vi "initalize delta(SubVI).vi"(9 "字符串":string, 11 "队列输出":refnum<queue>) -> ()   [LabVIEW 2019, in "SubVI.lvlib"]
uses:
  SubVI.lvlib
  lib/Keithley 622x/Configure/Delta PDelta DCon Modes/Typedefs/KE622x -- Delta Mode Params.ctl
  lib/Keithley 622x/Configure/Delta PDelta DCon Modes/Low Level/Typedefs/KE622x -- Delta PDelta Mode High Level.ctl
  lib/Keithley 622x/Configure/Delta PDelta DCon Modes/Low Level/Typedefs/KE622x -- Delta PDelta Mode Low Level.ctl
  lib/Keithley 622x/Configure/Delta PDelta DCon Modes/Low Level/Typedefs/KE622x -- Delta DCon Mode Delay.ctl
  lib/Keithley 622x/Configure/Delta PDelta DCon Modes/Low Level/Typedefs/KE622x -- Delta PDelta Mode Num Cycles Mode.ctl
  lib/Keithley 622x/Configure/Delta PDelta DCon Modes/Low Level/Typedefs/KE622x -- Delta PDelta Mode Num Cycles.ctl
  lib/Keithley 622x/Configure/2182 -A/Low Level/Typedefs/KE2182 -- Voltage Ranges.ctl
  lib/Keithley 622x/Configure/2182 -A/Low Level/Typedefs/KE2182 -- Filter Type.ctl
  lib/Keithley 622x/Configure/2182 -A/Low Level/Typedefs/KE2182 -- Filter Count.ctl
  lib/Keithley 622x/Configure/2182 -A/Low Level/Typedefs/KE2182 -- Filter Window.ctl
  lib/Keithley 622x/Configure/2182 -A/Low Level/Typedefs/KE2182 -- NPLCs.ctl
  config.ctl
  Instrument.ctl
  lib/QDInstrument.dll
  <vilib>/NI/Modbus Library/API/Master/Modbus Master.lvclass
  lib/Keithley 622x/Configure/Units/Typedefs/KE622x -- Voltage Meas Units.ctl
  lib/Keithley 622x/Keithley 622x.lvlib
panel:
  in  "2812 -A Params In":T6={"Auto Range?"=FALSE, "Man / Selected\nRange"=enum."10mV", "Enable Digital\nFilter?"=FALSE, "Filter Type"=enum."Moving", "Filter Count"=10, "Filter\nWindow (%)"=0.01, "Enable Analog\nFilter?"=FALSE, "NPLCs"=5} {"Filter\nWindow (%)" min=0.0 max=10.0 step=0.01 format="%.2f"; "Filter Count" min=1 max=100; "NPLCs" min=1 max=10}
  in  "Delta Mode Params In":T7={"High Level (A)"=0.001, "Low Level (A)"=-0.001, "Delay (s)"=0.002, "Num Cycles Mode"=enum."Finite Count", "Finite Count"=1, "Abort On\nCompliance?"=FALSE, "Cold Swithing\nMode Enabled?"=FALSE} {"Finite Count" min=1 max=65536; "Low Level (A)" min=-0.105 max=0.0 format="%.3p"; "High Level (A)" min=0.0 max=0.105 format="%.3p"; "Delay (s)" min=0.001 max=9999.999 format="%.3f"}
  in  "6221 Resource":refnum<visa-resource-name>="GPIB0::24::INSTR"
  # "(真是通道1，假是通道2)"
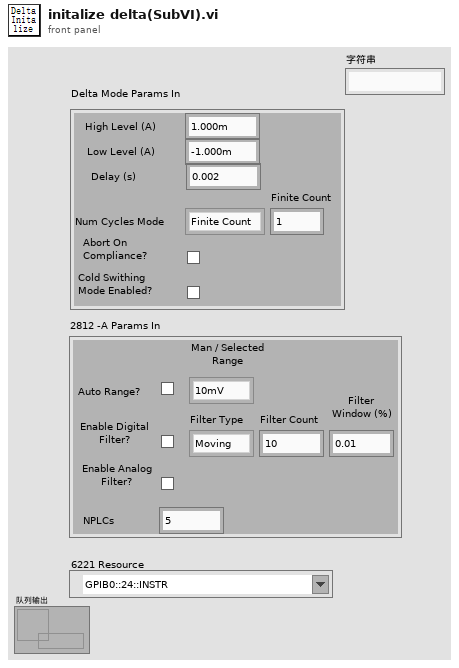
[diagram p1: front panel]
types:
  T1 = typedef "Keithley 622x.lvlib/KE2182 -- Voltage Ranges.ctl" = enum16{"10mV", "100mV", "1V", "10V", "100V"}
  T2 = typedef "Keithley 622x.lvlib/KE2182 -- Filter Type.ctl" = enum16{"Moving", "Repeat"}
  T3 = typedef "Keithley 622x.lvlib/KE2182 -- Filter Count.ctl" = u32
  T4 = typedef "Keithley 622x.lvlib/KE2182 -- Filter Window.ctl" = dbl
  T5 = typedef "Keithley 622x.lvlib/KE2182 -- NPLCs.ctl" = u32
  T6 = cluster{"Auto Range?":bool, "Man / Selected\nRange":T1, "Enable Digital\nFilter?":bool, "Filter Type":T2, "Filter Count":T3, "Filter\nWindow (%)":T4, "Enable Analog\nFilter?":bool, "NPLCs":T5}
  T7 = typedef "Keithley 622x.lvlib/KE622x -- Delta Mode Params.ctl" = cluster{"High Level (A)":T8, "Low Level (A)":T9, "Delay (s)":T10, "Num Cycles Mode":T11, "Finite Count":T12, "Abort On\nCompliance?":bool, "Cold Swithing\nMode Enabled?":bool}
  T8 = typedef "Keithley 622x.lvlib/KE622x -- Delta PDelta Mode High Level.ctl" = dbl
  T9 = typedef "Keithley 622x.lvlib/KE622x -- Delta PDelta Mode Low Level.ctl" = dbl
  T10 = typedef "Keithley 622x.lvlib/KE622x -- Delta DCon Mode Delay.ctl" = dbl
  T11 = typedef "Keithley 622x.lvlib/KE622x -- Delta PDelta Mode Num Cycles Mode.ctl" = enum16{"Finite Count", "Infinite"}
  T12 = typedef "Keithley 622x.lvlib/KE622x -- Delta PDelta Mode Num Cycles.ctl" = u32
  T13 = typedef "Keithley 622x.lvlib/KE622x -- Voltage Meas Units.ctl" = enum16{"Volts", "Ohms", "Watts", "Siemens"}
  T14 = typedef "config.ctl" = cluster{"initialize":string, "6221":cluster{"6221 Resource":refnum<visa-resource-name>, "Delta status":bool}, "7001":cluster{"Ch":bool}, "SR830+6221":cluster{"source":u16, "阻抗":dbl, "量程入 4":i32, "量程入 3":i32, "量程入 2":i32, "量程入 1":i32, "电流":dbl, "SR830 2":bool, "SR830 3":bool, "SR830 4":bool, "SR830 1":bool, "VISA 1":refnum<visa-resource-name>, "VISA 2":refnum<visa-resource-name>, "VISA 3":refnum<visa-resource-name>, "VISA 4":refnum<visa-resource-name>, "量程":enum16{"量程每次测量会判定", "量程不变为设定值"}}, "2400":cluster{"2400":bool, "VISA":refnum<visa-resource-name>}, "ch":cluster{"ch str":string, "ch1":bool, "ch2":bool, "布尔":bool}, "error":bool, "数据文件路径":path, "log":cluster{"log路径":path, "log interval":dbl}, "Instrument":T15}
  T15 = typedef "Instrument.ctl" = cluster{"335 Resource":refnum<visa-resource-name>, "Input (0:A)":u16, "Instrument Type":i32, "quantum design":refnum<k24>, "Heater Output (1:1)":u16, "335state":refnum<vi>, "semaphore":T16, "TCP master instance":refnum<class "Modbus Master.lvclass">}
  T16 = typedef "Semaphore RefNum" = refnum<k1>
  T17 = typedef "Keithley 622x.lvlib/KE622x -- On Off Control.ctl" = enum16{"Off", "On"}
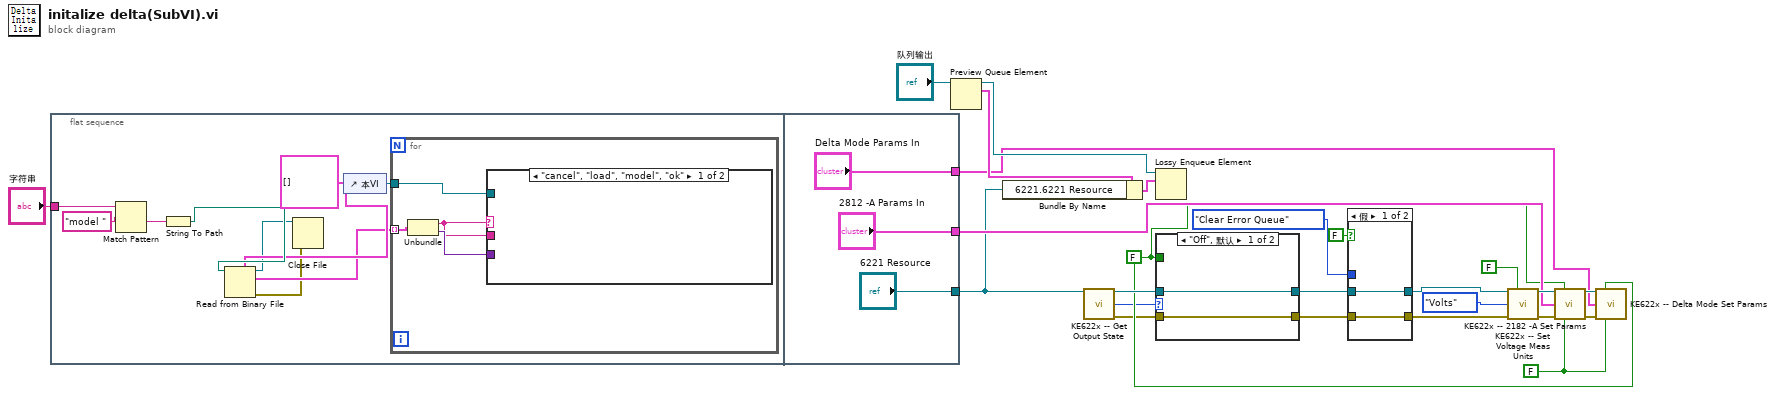
[diagram p0: block diagram]
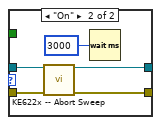
[diagram p2: hidden frame]
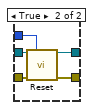
[diagram p3: hidden frame]
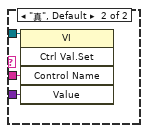
[diagram p4: hidden frame]
diagram:
  w15 = FALSE
  w6 = FALSE
  n1 = flat-sequence {
    tunnel: "字符串" -> [w34]
    tunnel: ["Delta Mode Params In"] -> w11
    tunnel: ["6221 Resource"] -> w5
    tunnel: ["2812 -A Params In"] -> w12
    frame #0 {
      n2 = Match Pattern(string=w34, regular expression="model " ("正则表达式")) -> (after substring=w33:string)  [unwired: 1 in, 3 out]
      n3 = String To Path(string=w33) -> (path=w30:path)
      n4 = Read from Binary File(5:cluster{"Name":string, "Variant Data":variant}[] [] ("控件值:获取全部"), 11:w30) -> (0:w26:errorcluster, 2:w28:cluster{"Name":string, "Variant Data":variant}[], 3:w27:refnum<file>)  [unwired: 4 in, 1 out]
      n5 = Close File(refnum=w27, error in=w26) -> ()  [unwired: 2 out]
      n6 = control-ref of="本VI"() -> (w31:refnum<vi>)
      n7 = for {
        tunnel: w28 -> [w38] mode=indexing
        tunnel: w31 -> [w37]
        n8 = Unbundle(w38) -> ("Name"=w35:string, "Variant Data"=w36:variant)
        n9 = case shown="\"cancel\", \"load\", \"model\", \"ok\"" w35 {
          tunnel: w37 -> [_ w41]
          tunnel: w35 -> [_ w40]
          tunnel: w36 -> [_ w39]
          frame "cancel", "load", "model", "ok" {
          }
          frame "真", Default {
            n10 = invoke class="VI" method="Ctrl Val.Set"(reference=w41, "Control Name"=w40, "Value"=w39) -> ()  [unwired: 2 in, 5 out]
          }
        }
      }
    }
    frame #1 {
    }
  }
  n11 = Preview Queue Element(queue="队列输出") -> (queue out=w22:refnum<queue>, element=w23:T14)  [unwired: 2 in, 2 out]
  n12 = Bundle By Name(cluster=w23, "6221.6221 Resource"=w5) -> (w21:T14)
  n13 = call "KE622x -- Get Output State.vi"("Resource In"=w5) -> ("Resource Out (dupl)"=w7:refnum<visa-resource-name>, "Output State"=w1:T17, "error out"=w3:errorcluster)  [unwired: 12 in]
  n14 = Lossy Enqueue Element(queue=w22, element=w21) -> ()  [unwired: 1 in, 4 out]
  n15 = case shown="\"Off\", 默认" w1 {
    tunnel: w7 -> [w46 w50]
    tunnel: w6 -> [_ _]
    tunnel: [w46 w49] -> w4
    tunnel: w3 -> [w45 w48]
    tunnel: [w45 w47] -> w2
    frame "Off", Default {
    }
    frame "On" {
      n16 = call "KE622x -- Abort Sweep.vi"("Resource In"=w50, "error in (no error)"=w48) -> ("Resource Out (dupl)"=w49:refnum<visa-resource-name>, "error out"=w47:errorcluster)  [unwired: 12 in]
      n17 = Wait (ms)(milliseconds to wait=u32 3000 ("等待时间（毫秒）")) -> ()  [unwired: 1 out]
    }
  }
  n18 = case shown="假" FALSE {
    tunnel: w4 -> [w53 w58]
    tunnel: enum16{"Clear Error Queue", "Error Query"}."Clear Error Queue" ("Error Queue Option") -> [_ w57]
    tunnel: [w53 w56] -> w19
    tunnel: w2 -> [w52 w55]
    tunnel: [w52 w54] -> w10
    frame False {
    }
    frame True {
      n19 = call "Reset.vi"("VISA resource name"=w58, "Error Queue Option"=w57, "error in (no error)"=w55) -> ("VISA resource name out"=w56:refnum<visa-resource-name>, "error out"=w54:errorcluster)  [unwired: 11 in]
    }
  }
  n20 = call "KE622x -- Set Voltage Meas Units.vi"("Resource In"=w19, "Check For SCPI Errors? (T)"=FALSE, "Voltage Meas Units"=KE622x_--_Voltage_Meas_Units."Volts", "error in (no error)"=w10) -> ("Resource Out (dupl)"=w20:refnum<visa-resource-name>, "error out"=w9:errorcluster)  [unwired: 10 in]
  n21 = call "KE622x -- 2182 -A Set Params.vi"("622x Resource In"=w20, "Check For SCPI Errors? (T)"=w6, "2812 -A Params In"=w12, "error in (no error)"=w9, "Read Back Set Values? (T)"=w15) -> ("622x Resource Out (dupl)"=w18:refnum<visa-resource-name>, "error out"=w8:errorcluster)  [unwired: 8 in, 1 out]
  n22 = call "KE622x -- Delta Mode Set Params.vi"("Resource In"=w18, "Check For SCPI Errors? (T)"=w6, "Delta Mode Params In"=w11, "error in (no error)"=w8, "Read Back Set Values? (T)"=w15) -> ()  [unwired: 8 in, 3 out]
